vi "Serial Read on Two Ports.vi"() -> ()   [LabVIEW 2021]
doc: "This example opens two VISA resources and configures one COM port to perform a write operation and the other COM port to perform a read operation. This VI will wait until the specified number of bytes is received at the port or until a termination character is read.\n\nThis example allows you perform diagnostic tests on your ports. You can use this example to perform a wrap-back test. Both serial ports must have the same basic configuration parameters. You can connect two of the ports using a null modem cable, which effectively connects one port's RX lines to the other port's TX lines. If you use a straight-through cable, one port's RX lines will be connected to the other port's RX lines, and you cannot communicate between the two ports."
uses:
  <vilib>/Instr/_visa.llb/VISA Configure Serial Port (Instr).vi
panel:
  out "XY Graph":cluster{"X":dbl, "Y":dbl}[](graph)
  in  "save":bool
  out "Waveform X":dbl(graph)
  out "Waveform Y":dbl(graph)
  out "Read String X":string
  in  "stop":bool
  out "Read String Y":string
  in  "VISA Resource Y":refnum<visa-resource-name>="COM2"
  in  "VISA Resource X":refnum<visa-resource-name>="COM1"
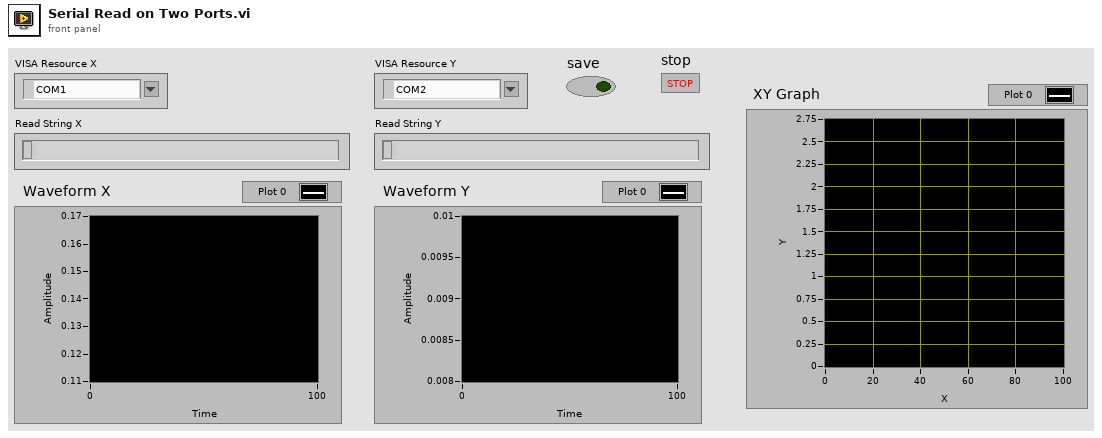
[diagram p1: front panel]
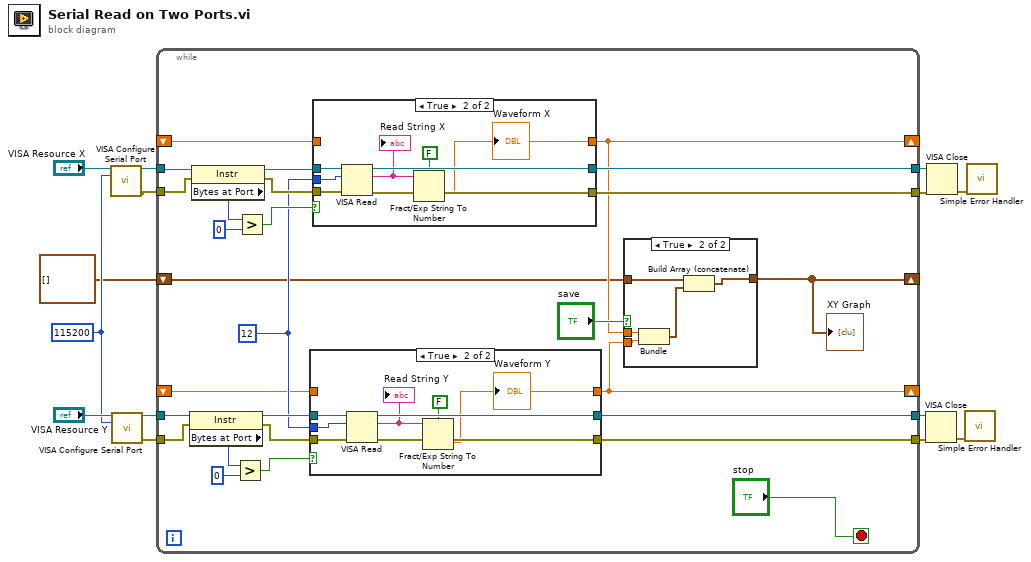
[diagram p0: block diagram]
diagram:
  w4 = u32 115200 ("baud rate (9600)")
  n1 = call-poly "VISA Configure Serial Port"("VISA resource name"="VISA Resource X", "baud rate (9600)"=w4) -> ("VISA resource name out"=w3:refnum<visa-resource-name>, "error out"=w12:errorcluster)  [unwired: 7 in, 5 out]
  n2 = call-poly "VISA Configure Serial Port"("VISA resource name"="VISA Resource Y", "baud rate (9600)"=w4) -> ("VISA resource name out"=w2:refnum<visa-resource-name>, "error out"=w5:errorcluster)  [unwired: 7 in, 5 out]
  n3 = while {
    tunnel: w2 -> [w36]
    tunnel: w3 -> [w29]
    tunnel: w5 -> [w34]
    tunnel: w12 -> [w27]
    tunnel: [w40] -> w10
    tunnel: [w39] -> w8
    tunnel: [w38] -> w7
    tunnel: [w37] -> w6
    shift-right: [w18] -> _
    shift-left: _ -> [w21]
    shift-right: [w17] -> _
    shift-left: _ -> [w20]
    shift-right: [w15] -> _
    shift-left: cluster{dbl, dbl}[] [] -> [w16]
    stop <- "stop" stop-if-true
    w22 = 12
    n4 = property class="Instr"(reference=w36, error in=w34) -> (reference out=w35:refnum<visa-resource-name>, error out=w33:errorcluster, "Bytes at Port"=w24:u32)
    n5 = property class="Instr"(reference=w29, error in=w27) -> (reference out=w28:refnum<visa-resource-name>, error out=w26:errorcluster, "Bytes at Port"=w23:u32)
    n6 = Greater?(x=w24, y=u32 0) -> (0:w31:bool)
    n7 = Greater?(x=w23, y=u32 0) -> (0:w25:bool)
    n8 = case shown="True" w31 {
      tunnel: w35 -> [w50 w58]
      tunnel: w33 -> [w49 w57]
      tunnel: [w49 w56] -> w39
      tunnel: [w50 w55] -> w38
      tunnel: w22 -> [_ w54]
      tunnel: [w48 w51] -> w17
      tunnel: w20 -> [w48 _]
      frame False {
      }
      frame True {
        n9 = VISA Read(VISA resource name=w58, byte count=w54, error in (no error)=w57) -> (VISA resource name out=w55:refnum<visa-resource-name>, read buffer=w53:string, error out=w56:errorcluster)  [unwired: 1 out]
        "Read String Y" <- w53
        n10 = Fract/Exp String To Number(use system decimal point (T)=FALSE, string=w53) -> (number=w51:dbl)  [unwired: 2 in, 1 out]
        "Waveform Y" <- w51
      }
    }
    n11 = case shown="True" w25 {
      tunnel: w28 -> [w60 w69]
      tunnel: w26 -> [w61 w68]
      tunnel: [w61 w67] -> w40
      tunnel: [w60 w66] -> w37
      tunnel: w22 -> [_ w65]
      tunnel: w21 -> [w59 _]
      tunnel: [w59 w62] -> w18
      frame False {
      }
      frame True {
        n12 = VISA Read(VISA resource name=w69, byte count=w65, error in (no error)=w68) -> (VISA resource name out=w66:refnum<visa-resource-name>, read buffer=w64:string, error out=w67:errorcluster)  [unwired: 1 out]
        "Read String X" <- w64
        n13 = Fract/Exp String To Number(use system decimal point (T)=FALSE, string=w64) -> (number=w62:dbl)  [unwired: 2 in, 1 out]
        "Waveform X" <- w62
      }
    }
    n14 = case shown="True" "save" {
      tunnel: w18 -> [_ w47]
      tunnel: w17 -> [_ w46]
      tunnel: w16 -> [w42 w44]
      tunnel: [w42 w43] -> w15
      frame False {
      }
      frame True {
        n15 = Bundle(w47, w46) -> (w45:cluster{dbl, dbl})  [unwired: 1 in]
        n16 = Build Array (concatenate)(w44, w45) -> (w43:cluster{dbl, dbl}[])
      }
    }
    "XY Graph" <- w15
  }
  n17 = VISA Close(VISA resource name=w7, error in (no error)=w8) -> (error out=w9:errorcluster)
  n18 = VISA Close(VISA resource name=w6, error in (no error)=w10) -> (error out=w11:errorcluster)
  n19 = call <vilib>:"Simple Error Handler.vi"("error in (no error)"=w9) -> ()  [unwired: 1 in, 8 out]
  n20 = call <vilib>:"Simple Error Handler.vi"("error in (no error)"=w11) -> ()  [unwired: 4 in, 5 out]
